vi "QR Factorization.vi"   [LabVIEW 2020, in "NI_AALPro.lvlib"]
doc: "LabVIEW no longer supports this VI. Use the QR Decomposition VI instead.\nPerforms the QR factorization of <B>A</B>. You can use this polymorphic VI to perform QR factorization on a real matrix or a complex matrix. The data type you wire to the <B>A</B> input determines the polymorphic instance to use.\nQR factorization is also called orthogonal-triangular factorization. The QR Factorization VI factors matrix <B>A</B> so that <B>A</B> = <B>QR</B>. You can use QR factorization to solve linear systems with more equations than unknowns."
uses:
  NI_AALPro.lvlib
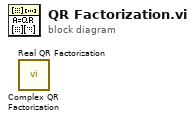
[diagram p0: block diagram]
diagram:
  n1 = call "Complex QR Factorization.vi"() -> ()  [unwired: 2 in, 3 out]
  n2 = call "Real QR Factorization.vi"() -> ()  [unwired: 2 in, 3 out]
